vi "test TCX read (installed 71).vi"() -> ()   [LabVIEW 2011] (continued)
tensions></Trackpoint><Trackpoint><Time>2008-03-03T23:09:45Z</Time><Position><LatitudeDegrees>35.861013</LatitudeDegrees><LongitudeDegrees>-78.894979</LongitudeDegrees></Position><AltitudeMeters>65.026</AltitudeMeters><DistanceMeters>13506.518</DistanceMeters><Cadence>82</Cadence><Extensions><TPX xmlns=\"http://www.garmin.com/xmlschemas/ActivityExtension/v2\"><Watts>176</Watts></TPX></Extensions></Trackpoint><Trackpoint><Time>2008-03-03T23:09:46Z</Time><Position><LatitudeDegrees>35.861010</LatitudeDegrees><LongitudeDegrees>-78.895077</LongitudeDegrees></Position><AltitudeMeters>65.988</AltitudeMeters><DistanceMeters>13515.292</DistanceMeters><Cadence>82</Cadence><Extensions><TPX xmlns=\"http://www.garmin.com/xmlschemas/ActivityExtension/v2\"><Watts>178</Watts></TPX></Extensions></Trackpoint><Trackpoint><Time>2008-03-03T23:09:47Z</Time><Position><LatitudeDegrees>35.861009</LatitudeDegrees><LongitudeDegrees>-78.895172</LongitudeDegrees></Position><AltitudeMeters>65.988</AltitudeMeters><DistanceMeters>13523.903</DistanceMeters><Cadence>79</Cadence><Extensions><TPX xmlns=\"http://www.garmin.com/xmlschemas/ActivityExtension/v2\"><Watts>351</Watts></TPX></Extensions></Trackpoint><Trackpoint><Time>2008-03-03T23:09:48Z</Time><Position><LatitudeDegrees>35.861007</LatitudeDegrees><LongitudeDegrees>-78.895264</LongitudeDegrees></Position><AltitudeMeters>66.468</AltitudeMeters><DistanceMeters>13532.188</DistanceMeters><Cadence>78</Cadence><Extensions><TPX xmlns=\"http://www.garmin.com/xmlschemas/ActivityExtension/v2\"><Watts>435</Watts></TPX></Extensions></Trackpoint><Trackpoint><Time>2008-03-03T23:09:49Z</Time><Position><LatitudeDegrees>35.861004</LatitudeDegrees><LongitudeDegrees>-78.895353</LongitudeDegrees></Position><AltitudeMeters>66.468</AltitudeMeters><DistanceMeters>13540.193</DistanceMeters><Cadence>74</Cadence><Extensions><TPX xmlns=\"http://www.garmin.com/xmlschemas/ActivityExtension/v2\"><Watts>444</Watts></TPX></Extensions></Trackpoint><Trackpoint><Time>2008-03-03T23:09:50Z</Time><Position><LatitudeDegrees>35.861000</LatitudeDegrees><LongitudeDegrees>-78.895439</LongitudeDegrees></Position><AltitudeMeters>67.430</AltitudeMeters><DistanceMeters>13547.961</DistanceMeters><Cadence>73</Cadence><Extensions><TPX xmlns=\"http://www.garmin.com/xmlschemas/ActivityExtension/v2\"><Watts>439</Watts></TPX></Extensions></Trackpoint><Trackpoint><Time>2008-03-03T23:09:51Z</Time><Position><LatitudeDegrees>35.860996</LatitudeDegrees><LongitudeDegrees>-78.895523</LongitudeDegrees></Position><AltitudeMeters>67.910</AltitudeMeters><DistanceMeters>13555.550</DistanceMeters><Cadence>71</Cadence><Extensions><TPX xmlns=\"http://www.garmin.com/xmlschemas/ActivityExtension/v2\"><Watts>436</Watts></TPX></Extensions></Trackpoint><Trackpoint><Time>2008-03-03T23:09:52Z</Time><Position><LatitudeDegrees>35.860994</LatitudeDegrees><LongitudeDegrees>-78.895604</LongitudeDegrees></Position><AltitudeMeters>68.391</AltitudeMeters><DistanceMeters>13562.899</DistanceMeters><Cadence>69</Cadence><Extensions><TPX xmlns=\"http://www.garmin.com/xmlschemas/ActivityExtension/v2\"><Watts>446</Watts></TPX></Extensions></Trackpoint><Trackpoint><Time>2008-03-03T23:09:53Z</Time><Position><LatitudeDegrees>35.860992</LatitudeDegrees><LongitudeDegrees>-78.895685</LongitudeDegrees></Position><AltitudeMeters>68.872</AltitudeMeters><DistanceMeters>13570.170</DistanceMeters><Cadence>69</Cadence><Extensions><TPX xmlns=\"http://www.garmin.com/xmlschemas/ActivityExtension/v2\"><Watts>446</Watts></TPX></Extensions></Trackpoint><Trackpoint><Time>2008-03-03T23:09:54Z</Time><Position><LatitudeDegrees>35.860991</LatitudeDegrees><LongitudeDegrees>-78.895764</LongitudeDegrees></Position><AltitudeMeters>68.872</AltitudeMeters><DistanceMeters>13577.373</DistanceMeters><Cadence>66</Cadence><Extensions><TPX xmlns=\"http://www.garmin.com/xmlschemas/ActivityExtension/v2\"><Watts>426</Watts></TPX></Extensions></Trackpoint><Trackpoint><Time>2008-03-03T23:09:55Z</Time><Position><LatitudeDegrees>35.860992</LatitudeDegrees><LongitudeDegrees>-78.895843</LongitudeDegrees></Position><AltitudeMeters>69.352</AltitudeMeters><DistanceMeters>13584.441</DistanceMeters><Cadence>66</Cadence><Extensions><TPX xmlns=\"http://www.garmin.com/xmlschemas/ActivityExtension/v2\"><Watts>423</Watts></TPX></Extensions></Trackpoint><Trackpoint><Time>2008-03-03T23:09:56Z</Time><Position><LatitudeDegrees>35.860994</LatitudeDegrees><LongitudeDegrees>-78.895919</LongitudeDegrees></Position><AltitudeMeters>69.352</AltitudeMeters><DistanceMeters>13591.366</DistanceMeters><Cadence>64</Cadence><Extensions><TPX xmlns=\"http://www.garmin.com/xmlschemas/ActivityExtension/v2\"><Watts>377</Watts></TPX></Extensions></Trackpoint><Trackpoint><Time>2008-03-03T23:09:57Z</Time><Position><LatitudeDegrees>35.860996</LatitudeDegrees><LongitudeDegrees>-78.895995</LongitudeDegrees></Position><AltitudeMeters>69.833</AltitudeMeters><DistanceMeters>13598.160</DistanceMeters><Cadence>63</Cadence><Extensions><TPX xmlns=\"http://www.garmin.com/xmlschemas/ActivityExtension/v2\"><Watts>379</Watts></TPX></Extensions></Trackpoint><Trackpoint><Time>2008-03-03T23:09:58Z</Time><Position><LatitudeDegrees>35.861001</LatitudeDegrees><LongitudeDegrees>-78.896070</LongitudeDegrees></Position><AltitudeMeters>70.794</AltitudeMeters><DistanceMeters>13604.948</DistanceMeters><Cadence>63</Cadence><Extensions><TPX xmlns=\"http://www.garmin.com/xmlschemas/ActivityExtension/v2\"><Watts>379</Watts></TPX></Extensions></Trackpoint><Trackpoint><Time>2008-03-03T23:09:59Z</Time><Position><LatitudeDegrees>35.861008</LatitudeDegrees><LongitudeDegrees>-78.896144</LongitudeDegrees></Position><AltitudeMeters>70.794</AltitudeMeters><DistanceMeters>13611.671</DistanceMeters><Cadence>62</Cadence><Extensions><TPX xmlns=\"http://www.garmin.com/xmlschemas/ActivityExtension/v2\"><Watts>421</Watts></TPX></Extensions></Trackpoint><Trackpoint><Time>2008-03-03T23:10:00Z</Time><Position><LatitudeDegrees>35.861015</LatitudeDegrees><LongitudeDegrees>-78.896216</LongitudeDegrees></Position><AltitudeMeters>71.275</AltitudeMeters><DistanceMeters>13618.257</DistanceMeters><Cadence>62</Cadence><Extensions><TPX xmlns=\"http://www.garmin.com/xmlschemas/ActivityExtension/v2\"><Watts>418</Watts></TPX></Extensions></Trackpoint><Trackpoint><Time>2008-03-03T23:10:01Z</Time><Position><LatitudeDegrees>35.861021</LatitudeDegrees><LongitudeDegrees>-78.896289</LongitudeDegrees></Position><AltitudeMeters>71.755</AltitudeMeters><DistanceMeters>13624.921</DistanceMeters><Cadence>62</Cadence><Extensions><TPX xmlns=\"http://www.garmin.com/xmlschemas/ActivityExtension/v2\"><Watts>394</Watts></TPX></Extensions></Trackpoint><Trackpoint><Time>2008-03-03T23:10:02Z</Time><Position><LatitudeDegrees>35.861026</LatitudeDegrees><LongitudeDegrees>-78.896364</LongitudeDegrees></Position><AltitudeMeters>72.236</AltitudeMeters><DistanceMeters>13631.681</DistanceMeters><Cadence>63</Cadence><Extensions><TPX xmlns=\"http://www.garmin.com/xmlschemas/ActivityExtension/v2\"><Watts>395</Watts></TPX></Extensions></Trackpoint><Trackpoint><Time>2008-03-03T23:10:03Z</Time><Position><LatitudeDegrees>35.861030</LatitudeDegrees><LongitudeDegrees>-78.896439</LongitudeDegrees></Position><AltitudeMeters>72.236</AltitudeMeters><DistanceMeters>13638.502</DistanceMeters><Cadence>64</Cadence><Extensions><TPX xmlns=\"http://www.garmin.com/xmlschemas/ActivityExtension/v2\"><Watts>400</Watts></TPX></Extensions></Trackpoint><Trackpoint><Time>2008-03-03T23:10:04Z</Time><Position><LatitudeDegrees>35.861034</LatitudeDegrees><LongitudeDegrees>-78.896516</LongitudeDegrees></Position><AltitudeMeters>72.717</AltitudeMeters><DistanceMeters>13645.401</DistanceMeters><Cadence>64</Cadence><Extensions><TPX xmlns=\"http://www.garmin.com/xmlschemas/ActivityExtension/v2\"><Watts>409</Watts></TPX></Extensions></Trackpoint><Trackpoint><Time>2008-03-03T23:10:05Z</Time><Position><LatitudeDegrees>35.861039</LatitudeDegrees><LongitudeDegrees>-78.896593</LongitudeDegrees></Position><AltitudeMeters>72.717</AltitudeMeters><DistanceMeters>13652.380</DistanceMeters><Cadence>64</Cadence><Extensions><TPX xmlns=\"http://www.garmin.com/xmlschemas/ActivityExtension/v2\"><Watts>411</Watts></TPX></Extensions></Trackpoint><Trackpoint><Time>2008-03-03T23:10:06Z</Time><Position><LatitudeDegrees>35.861044</LatitudeDegrees><LongitudeDegrees>-78.896670</LongitudeDegrees></Position><AltitudeMeters>72.717</AltitudeMeters><DistanceMeters>13659.413</DistanceMeters><Cadence>67</Cadence><Extensions><TPX xmlns=\"http://www.garmin.com/xmlschemas/ActivityExtension/v2\"><Watts>418</Watts></TPX></Extensions></Trackpoint><Trackpoint><Time>2008-03-03T23:10:07Z</Time><Position><LatitudeDegrees>35.861050</LatitudeDegrees><LongitudeDegrees>-78.896750</LongitudeDegrees></Position><AltitudeMeters>73.198</AltitudeMeters><DistanceMeters>13666.635</DistanceMeters><Cadence>67</Cadence><Extensions><TPX xmlns=\"http://www.garmin.com/xmlschemas/ActivityExtension/v2\"><Watts>404</Watts></TPX></Extensions></Trackpoint><Trackpoint><Time>2008-03-03T23:10:08Z</Time><Position><LatitudeDegrees>35.861056</LatitudeDegrees><LongitudeDegrees>-78.896830</LongitudeDegrees></Position><AltitudeMeters>73.678</AltitudeMeters><DistanceMeters>13673.963</DistanceMeters><Cadence>69</Cadence><Extensions><TPX xmlns=\"http://www.garmin.com/xmlschemas/ActivityExtension/v2\"><Watts>388</Watts></TPX></Extensions></Trackpoint><Trackpoint><Time>2008-03-03T23:10:09Z</Time><Position><LatitudeDegrees>35.861062</LatitudeDegrees><LongitudeDegrees>-78.896912</LongitudeDegrees></Position><AltitudeMeters>74.159</AltitudeMeters><DistanceMeters>13681.418</DistanceMeters><Cadence>70</Cadence><Extensions><TPX xmlns=\"http://www.garmin.com/xmlschemas/ActivityExtension/v2\"><Watts>386</Watts></TPX></Extensions></Trackpoint><Trackpoint><Time>2008-03-03T23:10:10Z</Time><Position><LatitudeDegrees>35.861070</LatitudeDegrees><LongitudeDegrees>-78.896996</LongitudeDegrees></Position><AltitudeMeters>74.640</AltitudeMeters><DistanceMeters>13689.080</DistanceMeters><Cadence>70</Cadence><Extensions><TPX xmlns=\"http://www.garmin.com/xmlschemas/ActivityExtension/v2\"><Watts>384</Watts></TPX></Extensions></Trackpoint><Trackpoint><Time>2008-03-03T23:10:11Z</Time><Position><LatitudeDegrees>35.861077</LatitudeDegrees><LongitudeDegrees>-78.897082</LongitudeDegrees></Position><AltitudeMeters>74.640</AltitudeMeters><DistanceMeters>13696.857</DistanceMeters><Cadence>72</Cadence><Extensions><TPX xmlns=\"http://www.garmin.com/xmlschemas/ActivityExtension/v2\"><Watts>388</Watts></TPX></Extensions></Trackpoint><Trackpoint><Time>2008-03-03T23:10:12Z</Time><Position><LatitudeDegrees>35.861085</LatitudeDegrees><LongitudeDegrees>-78.897170</LongitudeDegrees></Position><AltitudeMeters>75.120</AltitudeMeters><DistanceMeters>13704.818</DistanceMeters><Cadence>74</Cadence><Extensions><TPX xmlns=\"http://www.garmin.com/xmlschemas/ActivityExtension/v2\"><Watts>392</Watts></TPX></Extensions></Trackpoint><Trackpoint><Time>2008-03-03T23:10:13Z</Time><Position><LatitudeDegrees>35.861095</LatitudeDegrees><LongitudeDegrees>-78.897259</LongitudeDegrees></Position><AltitudeMeters>75.601</AltitudeMeters><DistanceMeters>13712.946</DistanceMeters><Cadence>76</Cadence><Extensions><TPX xmlns=\"http://www.garmin.com/xmlschemas/ActivityExtension/v2\"><Watts>393</Watts></TPX></Extensions></Trackpoint><Trackpoint><Time>2008-03-03T23:10:14Z</Time><Position><LatitudeDegrees>35.861106</LatitudeDegrees><LongitudeDegrees>-78.897348</LongitudeDegrees></Position><AltitudeMeters>75.120</AltitudeMeters><DistanceMeters>13721.106</DistanceMeters><Cadence>75</Cadence><Extensions><TPX xmlns=\"http://www.garmin.com/xmlschemas/ActivityExtension/v2\"><Watts>364</Watts></TPX></Extensions></Trackpoint><Trackpoint><Time>2008-03-03T23:10:15Z</Time><Position><LatitudeDegrees>35.861116</LatitudeDegrees><LongitudeDegrees>-78.897436</LongitudeDegrees></Position><AltitudeMeters>75.601</AltitudeMeters><DistanceMeters>13729.120</DistanceMeters><Cadence>74</Cadence><Extensions><TPX xmlns=\"http://www.garmin.com/xmlschemas/ActivityExtension/v2\"><Watts>233</Watts></TPX></Extensions></Trackpoint><Trackpoint><Time>2008-03-03T23:10:16Z</Time><Position><LatitudeDegrees>35.861124</LatitudeDegrees><LongitudeDegrees>-78.897522</LongitudeDegrees></Position><AltitudeMeters>75.601</AltitudeMeters><DistanceMeters>13736.914</DistanceMeters><Cadence>72</Cadence><Extensions><TPX xmlns=\"http://www.garmin.com/xmlschemas/ActivityExtension/v2\"><Watts>107</Watts></TPX></Extensions></Trackpoint><Trackpoint><Time>2008-03-03T23:10:17Z</Time><Position><LatitudeDegrees>35.861136</LatitudeDegrees><LongitudeDegrees>-78.897604</LongitudeDegrees></Position><AltitudeMeters>75.601</AltitudeMeters><DistanceMeters>13744.367</DistanceMeters><Cadence>69</Cadence><Extensions><TPX xmlns=\"http://www.garmin.com/xmlschemas/ActivityExtension/v2\"><Watts>52</Watts></TPX></Extensions></Trackpoint><Trackpoint><Time>2008-03-03T23:10:18Z</Time><Position><LatitudeDegrees>35.861166</LatitudeDegrees><LongitudeDegrees>-78.897671</LongitudeDegrees></Position><AltitudeMeters>76.081</AltitudeMeters><DistanceMeters>13751.099</DistanceMeters><Cadence>68</Cadence><Extensions><TPX xmlns=\"http://www.garmin.com/xmlschemas/ActivityExtension/v2\"><Watts>52</Watts></TPX></Extensions></Trackpoint><Trackpoint><Time>2008-03-03T23:10:19Z</Time><Position><LatitudeDegrees>35.861226</LatitudeDegrees><LongitudeDegrees>-78.897707</LongitudeDegrees></Position><AltitudeMeters>76.562</AltitudeMeters><DistanceMeters>13758.359</DistanceMeters><Cadence>63</Cadence><Extensions><TPX xmlns=\"http://www.garmin.com/xmlschemas/ActivityExtension/v2\"><Watts>60</Watts></TPX></Extensions></Trackpoint><Trackpoint><Time>2008-03-03T23:10:20Z</Time><Position><LatitudeDegrees>35.861288</LatitudeDegrees><LongitudeDegrees>-78.897691</LongitudeDegrees></Position><AltitudeMeters>77.043</AltitudeMeters><DistanceMeters>13765.466</DistanceMeters><Cadence>63</Cadence><Extensions><TPX xmlns=\"http://www.garmin.com/xmlschemas/ActivityExtension/v2\"><Watts>59</Watts></TPX></Extensions></Trackpoint><Trackpoint><Time>2008-03-03T23:10:21Z</Time><Position><LatitudeDegrees>35.861350</LatitudeDegrees><LongitudeDegrees>-78.897655</LongitudeDegrees></Position><AltitudeMeters>77.043</AltitudeMeters><DistanceMeters>13773.082</DistanceMeters><Cadence>65</Cadence><Extensions><TPX xmlns=\"http://www.garmin.com/xmlschemas/ActivityExtension/v2\"><Watts>377</Watts></TPX></Extensions></Trackpoint><Trackpoint><Time>2008-03-03T23:10:22Z</Time><Position><LatitudeDegrees>35.861415</LatitudeDegrees><LongitudeDegrees>-78.897617</LongitudeDegrees></Position><AltitudeMeters>77.523</AltitudeMeters><DistanceMeters>13781.167</DistanceMeters><Cadence>68</Cadence><Extensions><TPX xmlns=\"http://www.garmin.com/xmlschemas/ActivityExtension/v2\"><Watts>429</Watts></TPX></Extensions></Trackpoint><Trackpoint><Time>2008-03-03T23:10:23Z</Time><Position><LatitudeDegrees>35.861477</LatitudeDegrees><LongitudeDegrees>-78.897576</LongitudeDegrees></Position><AltitudeMeters>77.523</AltitudeMeters><DistanceMeters>13788.905</DistanceMeters><Cadence>70</Cadence><Extensions><TPX xmlns=\"http://www.garmin.com/xmlschemas/ActivityExtension/v2\"><Watts>456</Watts></TPX></Extensions></Trackpoint><Trackpoint><Time>2008-03-03T23:10:24Z</Time><Position><LatitudeDegrees>35.861541</LatitudeDegrees><LongitudeDegrees>-78.897533</LongitudeDegrees></Position><AltitudeMeters>78.004</AltitudeMeters><DistanceMeters>13797.001</DistanceMeters><Cadence>71</Cadence><Extensions><TPX xmlns=\"http://www.garmin.com/xmlschemas/ActivityExtension/v2\"><Watts>430</Watts></TPX></Extensions></Trackpoint><Trackpoint><Time>2008-03-03T23:10:25Z</Time><Position><LatitudeDegrees>35.861605</LatitudeDegrees><LongitudeDegrees>-78.897493</LongitudeDegrees></Position><AltitudeMeters>78.004</AltitudeMeters><DistanceMeters>13804.948</DistanceMeters><Cadence>73</Cadence><Extensions><TPX xmlns=\"http://www.garmin.com/xmlschemas/ActivityExtension/v2\"><Watts>403</Watts></TPX></Extensions></Trackpoint><Trackpoint><Time>2008-03-03T23:10:26Z</Time><Position><LatitudeDegrees>35.861668</LatitudeDegrees><LongitudeDegrees>-78.897454</LongitudeDegrees></Position><AltitudeMeters>78.485</AltitudeMeters><DistanceMeters>13812.879</DistanceMeters><Cadence>73</Cadence><Extensions><TPX xmlns=\"http://www.garmin.com/xmlschemas/ActivityExtension/v2\"><Watts>345</Watts></TPX></Extensions></Trackpoint><Trackpoint><Time>2008-03-03T23:10:27Z</Time><Position><LatitudeDegrees>35.861733</LatitudeDegrees><LongitudeDegrees>-78.897415</LongitudeDegrees></Position><AltitudeMeters>78.004</AltitudeMeters><DistanceMeters>13820.811</DistanceMeters><Cadence>72</Cadence><Extensions><TPX xmlns=\"http://www.garmin.com/xmlschemas/ActivityExtension/v2\"><Watts>316</Watts></TPX></Extensions></Trackpoint><Trackpoint><Time>2008-03-03T23:10:28Z</Time><Position><LatitudeDegrees>35.861798</LatitudeDegrees><LongitudeDegrees>-78.897377</LongitudeDegrees></Position><AltitudeMeters>78.485</AltitudeMeters><DistanceMeters>13828.832</DistanceMeters><Cadence>72</Cadence><Extensions><TPX xmlns=\"http://www.garmin.com/xmlschemas/ActivityExtension/v2\"><Watts>292</Watts></TPX></Extensions></Trackpoint><Trackpoint><Time>2008-03-03T23:10:29Z</Time><Position><LatitudeDegrees>35.861861</LatitudeDegrees><LongitudeDegrees>-78.897341</LongitudeDegrees></Position><AltitudeMeters>78.965</AltitudeMeters><DistanceMeters>13836.527</DistanceMeters><Cadence>72</Cadence><Extensions><TPX xmlns=\"http://www.garmin.com/xmlschemas/ActivityExtension/v2\"><Watts>274</Watts></TPX></Extensions></Trackpoint><Trackpoint><Time>2008-03-03T23:10:30Z</Time><Position><LatitudeDegrees>35.861924</LatitudeDegrees><LongitudeDegrees>-78.897309</LongitudeDegrees></Position><AltitudeMeters>79.446</AltitudeMeters><DistanceMeters>13844.088</DistanceMeters><Cadence>72</Cadence><Extensions><TPX xmlns=\"http://www.garmin.com/xmlschemas/ActivityExtension/v2\"><Watts>276</Watts></TPX></Extensions></Trackpoint><Trackpoint><Time>2008-03-03T23:10:31Z</Time><Position><LatitudeDegrees>35.861985</LatitudeDegrees><LongitudeDegrees>-78.897277</LongitudeDegrees></Position><AltitudeMeters>79.446</AltitudeMeters><DistanceMeters>13851.475</DistanceMeters><Cadence>70</Cadence><Extensions><TPX xmlns=\"http://www.garmin.com/xmlschemas/ActivityExtension/v2\"><Watts>273</Watts></TPX></Extensions></Trackpoint><Trackpoint><Time>2008-03-03T23:10:32Z</Time><Position><LatitudeDegrees>35.862050</LatitudeDegrees><LongitudeDegrees>-78.897251</LongitudeDegrees></Position><AltitudeMeters>79.446</AltitudeMeters><DistanceMeters>13859.048</DistanceMeters><Cadence>70</Cadence><Extensions><TPX xmlns=\"http://www.garmin.com/xmlschemas/ActivityExtension/v2\"><Watts>271</Watts></TPX></Extensions></Trackpoint><Trackpoint><Time>2008-03-03T23:10:33Z</Time><Position><LatitudeDegrees>35.862113</LatitudeDegrees><LongitudeDegrees>-78.897226</LongitudeDegrees></Position><AltitudeMeters>79.446</AltitudeMeters><DistanceMeters>13866.438</DistanceMeters><Cadence>69</Cadence><Extensions><TPX xmlns=\"http://www.garmin.com/xmlschemas/ActivityExtension/v2\"><Watts>260</Watts></TPX></Extensions></Trackpoint><Trackpoint><Time>2008-03-03T23:10:34Z</Time><Position><LatitudeDegrees>35.862177</LatitudeDegrees><LongitudeDegrees>-78.897201</LongitudeDegrees></Position><AltitudeMeters>79.927</AltitudeMeters><DistanceMeters>13873.806</DistanceMeters><Cadence>68</Cadence><Extensions><TPX xmlns=\"http://www.garmin.com/xmlschemas/ActivityExtension/v2\"><Watts>233</Watts></TPX></Extensions></Trackpoint><Trackpoint><Time>2008-03-03T23:10:35Z</Time><Position><LatitudeDegrees>35.862241</LatitudeDegrees><LongitudeDegrees>-78.897177</LongitudeDegrees></Position><AltitudeMeters>79.927</AltitudeMeters><DistanceMeters>13881.198</DistanceMeters><Cadence>68</Cadence><Extensions><TPX xmlns=\"http://www.garmin.com/xmlschemas/ActivityExtension/v2\"><Watts>232</Watts></TPX></Extensions></Trackpoint><Trackpoint><Time>2008-03-03T23:10:36Z</Time><Position><LatitudeDegrees>35.862304</LatitudeDegrees><LongitudeDegrees>-78.897157</LongitudeDegrees></Position><AltitudeMeters>79.927</AltitudeMeters><DistanceMeters>13888.406</DistanceMeters><Cadence>67</Cadence><Extensions><TPX xmlns=\"http://www.garmin.com/xmlschemas/ActivityExtension/v2\"><Watts>164</Watts></TPX></Extensions></Trackpoint><Trackpoint><Time>2008-03-03T23:10:37Z</Time><Position><LatitudeDegrees>35.862367</LatitudeDegrees><LongitudeDegrees>-78.897137</LongitudeDegrees></Position><AltitudeMeters>80.407</AltitudeMeters><DistanceMeters>13895.671</DistanceMeters><Cadence>66</Cadence><Extensions><TPX xmlns=\"http://www.garmin.com/xmlschemas/ActivityExtension/v2\"><Watts>164</Watts></TPX></Extensions></Trackpoint><Trackpoint><Time>2008-03-03T23:10:38Z</Time><Position><LatitudeDegrees>35.862429</LatitudeDegrees><LongitudeDegrees>-78.897119</LongitudeDegrees></Position><AltitudeMeters>80.407</AltitudeMeters><DistanceMeters>13902.797</DistanceMeters><Cadence>66</Cadence><Extensions><TPX xmlns=\"http://www.garmin.com/xmlschemas/ActivityExtension/v2\"><Watts>171</Watts></TPX></Extensions></Trackpoint><Trackpoint><Time>2008-03-03T23:10:39Z</Time><Position><LatitudeDegrees>35.862493</LatitudeDegrees><LongitudeDegrees>-78.897101</LongitudeDegrees></Position><AltitudeMeters>80.407</AltitudeMeters><DistanceMeters>13910.059</DistanceMeters><Cadence>66</Cadence><Extensions><TPX xmlns=\"http://www.garmin.com/xmlschemas/ActivityExtension/v2\"><Watts>173</Watts></TPX></Extensions></Trackpoint><Trackpoint><Time>2008-03-03T23:10:40Z</Time><Position><LatitudeDegrees>35.862555</LatitudeDegrees><LongitudeDegrees>-78.897088</LongitudeDegrees></Position><AltitudeMeters>80.407</AltitudeMeters><DistanceMeters>13917.023</DistanceMeters><Cadence>66</Cadence><Extensions><TPX xmlns=\"http://www.garmin.com/xmlschemas/ActivityExtension/v2\"><Watts>170</Watts></TPX></Extensions></Trackpoint><Trackpoint><Time>2008-03-03T23:10:41Z</Time><Position><LatitudeDegrees>35.862619</LatitudeDegrees><LongitudeDegrees>-78.897075</LongitudeDegrees></Position><AltitudeMeters>80.407</AltitudeMeters><DistanceMeters>13924.162</DistanceMeters><Cadence>66</Cadence><Extensions><TPX xmlns=\"http://www.garmin.com/xmlschemas/ActivityExtension/v2\"><Watts>163</Watts></TPX></Extensions></Trackpoint><Trackpoint><Time>2008-03-03T23:10:42Z</Time><Position><LatitudeDegrees>35.862684</LatitudeDegrees><LongitudeDegrees>-78.897063</LongitudeDegrees></Position><AltitudeMeters>80.888</AltitudeMeters><DistanceMeters>13931.451</DistanceMeters><Cadence>66</Cadence><Extensions><TPX xmlns=\"http://www.garmin.com/xmlschemas/ActivityExtension/v2\"><Watts>165</Watts></TPX></Extensions></Trackpoint><Trackpoint><Time>2008-03-03T23:10:43Z</Time><Position><LatitudeDegrees>35.862747</LatitudeDegrees><LongitudeDegrees>-78.897053</LongitudeDegrees></Position><AltitudeMeters>80.888</AltitudeMeters><DistanceMeters>13938.466</DistanceMeters><Cadence>65</Cadence><Extensions><TPX xmlns=\"http://www.garmin.com/xmlschemas/ActivityExtension/v2\"><Watts>145</Watts></TPX></Extensions></Trackpoint><Trackpoint><Time>2008-03-03T23:10:44Z</Time><Position><LatitudeDegrees>35.862810</LatitudeDegrees><LongitudeDegrees>-78.897044</LongitudeDegrees></Position><AltitudeMeters>80.888</AltitudeMeters><DistanceMeters>13945.525</DistanceMeters><Cadence>65</Cadence><Extensions><TPX xmlns=\"http://www.garmin.com/xmlschemas/ActivityExtension/v2\"><Watts>149</Watts></TPX></Extensions></Trackpoint><Trackpoint><Time>2008-03-03T23:10:45Z</Time><Position><LatitudeDegrees>35.862874</LatitudeDegrees><LongitudeDegrees>-78.897035</LongitudeDegrees></Position><AltitudeMeters>81.369</AltitudeMeters><DistanceMeters>13952.661</DistanceMeters><Cadence>65</Cadence><Extensions><TPX xmlns=\"http://www.garmin.com/xmlschemas/ActivityExtension/v2\"><Watts>137</Watts></TPX></Extensions></Trackpoint><Trackpoint><Time>2008-03-03T23:10:46Z</Time><Position><LatitudeDegrees>35.862936</LatitudeDegrees><LongitudeDegrees>-78.897027</LongitudeDegrees></Position><AltitudeMeters>81.369</AltitudeMeters><DistanceMeters>13959.629</DistanceMeters><Cadence>64</Cadence><Extensions><TPX xmlns=\"http://www.garmin.com/xmlschemas/ActivityExtension/v2\"><Watts>136</Watts></TPX></Extensions></Trackpoint><Trackpoint><Time>2008-03-03T23:10:47Z</Time><Position><LatitudeDegrees>35.862997</LatitudeDegrees><LongitudeDegrees>-78.897017</LongitudeDegrees></Position><AltitudeMeters>81.369</AltitudeMeters><DistanceMeters>13966.494</DistanceMeters><Cadence>65</Cadence><Extensions><TPX xmlns=\"http://www.garmin.com/xmlschemas/ActivityExtension/v2\"><Watts>138</Watts></TPX></Extensions></Trackpoint><Trackpoint><Time>2008-03-03T23:10:48Z</Time><Position><LatitudeDegrees>35.863060</LatitudeDegrees><LongitudeDegrees>-78.897006</LongitudeDegrees></Position><AltitudeMeters>81.369</AltitudeMeters><DistanceMeters>13973.530</DistanceMeters><Cadence>65</Cadence><Extensions><TPX xmlns=\"http://www.garmin.com/xmlschemas/ActivityExtension/v2\"><Watts>130</Watts></TPX></Extensions></Trackpoint><Trackpoint><Time>2008-03-03T23:10:49Z</Time><Position><LatitudeDegrees>35.863124</LatitudeDegrees><LongitudeDegrees>-78.896995</LongitudeDegrees></Position><AltitudeMeters>81.369</AltitudeMeters><DistanceMeters>13980.699</DistanceMeters><Cadence>65</Cadence><Extensions><TPX xmlns=\"http://www.garmin.com/xmlschemas/ActivityExtension/v2\"><Watts>126</Watts></TPX></Extensions></Trackpoint><Trackpoint><Time>2008-03-03T23:10:50Z</Time><Position><LatitudeDegrees>35.863189</LatitudeDegrees><LongitudeDegrees>-78.896986</LongitudeDegrees></Position><AltitudeMeters>81.849</AltitudeMeters><DistanceMeters>13987.968</DistanceMeters><Cadence>65</Cadence><Extensions><TPX xmlns=\"http://www.garmin.com/xmlschemas/ActivityExtension/v2\"><Watts>125</Watts></TPX></Extensions></Trackpoint><Trackpoint><Time>2008-03-03T23:10:51Z</Time><Position><LatitudeDegrees>35.863253</LatitudeDegrees><LongitudeDegrees>-78.896977</LongitudeDegrees></Position><AltitudeMeters>81.849</AltitudeMeters><DistanceMeters>13995.102</DistanceMeters><Cadence>65</Cadence><Extensions><TPX xmlns=\"http://www.garmin.com/xmlschemas/ActivityExtension/v2\"><Watts>105</Watts></TPX></Extensions></Trackpoint><Trackpoint><Time>2008-03-03T23:10:52Z</Time><Position><LatitudeDegrees>35.863315</LatitudeDegrees><LongitudeDegrees>-78.896968</LongitudeDegrees></Position><AltitudeMeters>81.849</AltitudeMeters><DistanceMeters>14001.995</DistanceMeters><Cadence>65</Cadence><Extensions><TPX xmlns=\"http://www.garmin.com/xmlschemas/ActivityExtension/v2\"><Watts>106</Watts></TPX></Extensions></Trackpoint><Trackpoint><Time>2008-03-03T23:10:53Z</Time><Position><LatitudeDegrees>35.863377</LatitudeDegrees><LongitudeDegrees>-78.896958</LongitudeDegrees></Position><AltitudeMeters>82.330</AltitudeMeters><DistanceMeters>14008.998</DistanceMeters><Cadence>65</Cadence><Extensions><TPX xmlns=\"http://www.garmin.com/xmlschemas/ActivityExtension/v2\"><Watts>99</Watts></TPX></Extensions></Trackpoint><Trackpoint><Time>2008-03-03T23:10:54Z</Time><Position><LatitudeDegrees>35.863440</LatitudeDegrees><LongitudeDegrees>-78.896948</LongitudeDegrees></Position><AltitudeMeters>82.330</AltitudeMeters><DistanceMeters>14015.998</DistanceMeters><Cadence>65</Cadence><Extensions><TPX xmlns=\"http://www.garmin.com/xmlschemas/ActivityExtension/v2\"><Watts>101</Watts></TPX></Extensions></Trackpoint><Trackpoint><Time>2008-03-03T23:10:55Z</Time><Position><LatitudeDegrees>35.863503</LatitudeDegrees><LongitudeDegrees>-78.896938</LongitudeDegrees></Position><AltitudeMeters>82.330</AltitudeMeters><DistanceMeters>14023.096</DistanceMeters><Cadence>65</Cadence><Extensions><TPX xmlns=\"http://www.garmin.com/xmlschemas/ActivityExtension/v2\"><Watts>100</Watts></TPX></Extensions></Trackpoint><Trackpoint><Time>2008-03-03T23:10:56Z</Time><Position><LatitudeDegrees>35.863566</LatitudeDegrees><LongitudeDegrees>-78.896934</LongitudeDegrees></Position><AltitudeMeters>82.330</AltitudeMeters><DistanceMeters>14030.051</DistanceMeters><Cadence>65</Cadence><Extensions><TPX xmlns=\"http://www.garmin.com/xmlschemas/ActivityExtension/v2\"><Watts>106</Watts></TPX></Extensions></Trackpoint><Trackpoint><Time>2008-03-03T23:10:57Z</Time><Position><LatitudeDegrees>35.863627</LatitudeDegrees><LongitudeDegrees>-78.896940</LongitudeDegrees></Position><AltitudeMeters>82.811</AltitudeMeters><DistanceMeters>14036.868</DistanceMeters><Cadence>64</Cadence><Extensions><TPX xmlns=\"http://www.garmin.com/xmlschemas/ActivityExtension/v2\"><Watts>106</Watts></TPX></Extensions></Trackpoint><Trackpoint><Time>2008-03-03T23:10:58Z</Time><Position><LatitudeDegrees>35.863685</LatitudeDegrees><LongitudeDegrees>-78.896964</LongitudeDegrees></Position><AltitudeMeters>83.291</AltitudeMeters><DistanceMeters>14043.521</DistanceMeters><Cadence>62</Cadence><Extensions><TPX xmlns=\"http://www.garmin.com/xmlschemas/ActivityExtension/v2\"><Watts>104</Watts></TPX></Extensions></Trackpoint><Trackpoint><Time>2008-03-03T23:10:59Z</Time><Position><LatitudeDegrees>35.863732</LatitudeDegrees><LongitudeDegrees>-78.897007</LongitudeDegrees></Position><AltitudeMeters>82.811</AltitudeMeters><DistanceMeters>14049.984</DistanceMeters><Cadence>62</Cadence><Extensions><TPX xmlns=\"http://www.garmin.com/xmlschemas/ActivityExtension/v2\"><Watts>102</Watts></TPX></Extensions></Trackpoint><Trackpoint><Time>2008-03-03T23:11:00Z</Time><Position><LatitudeDegrees>35.863767</LatitudeDegrees><LongitudeDegrees>-78.897066</LongitudeDegrees></Position><AltitudeMeters>83.291</AltitudeMeters><DistanceMeters>14056.616</DistanceMeters><Cadence>62</Cadence><Extensions><TPX xmlns=\"http://www.garmin.com/xmlschemas/ActivityExtension/v2\"><Watts>97</Watts></TPX></Extensions></Trackpoint><Trackpoint><Time>2008-03-03T23:11:01Z</Time><Position><LatitudeDegrees>35.863788</LatitudeDegrees><LongitudeDegrees>-78.897137</LongitudeDegrees></Position><AltitudeMeters>83.291</AltitudeMeters><DistanceMeters>14063.417</DistanceMeters><Cadence>64</Cadence><Extensions><TPX xmlns=\"http://www.garmin.com/xmlschemas/ActivityExtension/v2\"><Watts>92</Watts></TPX></Extensions></Trackpoint><Trackpoint><Time>2008-03-03T23:11:02Z</Time><Position><LatitudeDegrees>35.863794</LatitudeDegrees><LongitudeDegrees>-78.897215</LongitudeDegrees></Position><AltitudeMeters>82.811</AltitudeMeters><DistanceMeters>14070.526</DistanceMeters><Cadence>64</Cadence><Extensions><TPX xmlns=\"http://www.garmin.com/xmlschemas/ActivityExtension/v2\"><Watts>92</Watts></TPX></Extensions></Trackpoint><Trackpoint><Time>2008-03-03T23:11:03Z</Time><Position><LatitudeDegrees>35.863787</LatitudeDegrees><LongitudeDegrees>-78.897296</LongitudeDegrees></Position><AltitudeMeters>83.291</AltitudeMeters><DistanceMeters>14077.847</DistanceMeters><Cadence>66</Cadence><Extensions><TPX xmlns=\"http://www.garmin.com/xmlschemas/ActivityExtension/v2\"><Watts>87</Watts></TPX></Extensions></Trackpoint><Trackpoint><Time>2008-03-03T23:11:04Z</Time><Position><LatitudeDegrees>35.863773</LatitudeDegrees><LongitudeDegrees>-78.897378</LongitudeDegrees></Position><AltitudeMeters>82.811</AltitudeMeters><DistanceMeters>14085.448</DistanceMeters><Cadence>68</Cadence><Extensions><TPX xmlns=\"http://www.garmin.com/xmlschemas/ActivityExtension/v2\"><Watts>87</Watts></TPX></Extensions></Trackpoint><Trackpoint><Time>2008-03-03T23:11:05Z</Time><Position><LatitudeDegrees>35.863759</LatitudeDegrees><LongitudeDegrees>-78.897462</LongitudeDegrees></Position><AltitudeMeters>82.811</AltitudeMeters><DistanceMeters>14093.145</DistanceMeters><Cadence>70</Cadence><Extensions><TPX xmlns=\"http://www.garmin.com/xmlschemas/ActivityExtension/v2\"><Watts>86</Watts></TPX></Extensions></Trackpoint><Trackpoint><Time>2008-03-03T23:11:06Z</Time><Position><LatitudeDegrees>35.863746</LatitudeDegrees><LongitudeDegrees>-78.897548</LongitudeDegrees></Position><AltitudeMeters>82.811</AltitudeMeters><DistanceMeters>14101.066</DistanceMeters><Cadence>72</Cadence><Extensions><TPX xmlns=\"http://www.garmin.com/xmlschemas/ActivityExtension/v2\"><Watts>86</Watts></TPX></Extensions></Trackpoint><Trackpoint><Time>2008-03-03T23:11:07Z</Time><Position><LatitudeDegrees>35.863735</LatitudeDegrees><LongitudeDegrees>-78.897635</LongitudeDegrees></Position><AltitudeMeters>82.811</AltitudeMeters><DistanceMeters>14109.060</DistanceMeters><Cadence>72</Cadence><Extensions><TPX xmlns=\"http://www.garmin.com/xmlschemas/ActivityExtension/v2\"><Watts>86</Watts></TPX></Extensions></Trackpoint><Trackpoint><Time>2008-03-03T23:11:08Z</Time><Position><LatitudeDegrees>35.863720</LatitudeDegrees><LongitudeDegrees>-78.897725</LongitudeDegrees></Position><AltitudeMeters>82.811</AltitudeMeters><DistanceMeters>14117.366</DistanceMeters><Cadence>74</Cadence><Extensions><TPX xmlns=\"http://www.garmin.com/xmlschemas/ActivityExtension/v2\"><Watts>80</Watts></TPX></Extensions></Trackpoint><Trackpoint><Time>2008-03-03T23:11:09Z</Time><Position><LatitudeDegrees>35.863704</LatitudeDegrees><LongitudeDegrees>-78.897817</LongitudeDegrees></Position><AltitudeMeters>82.330</AltitudeMeters><DistanceMeters>14125.814</DistanceMeters><Cadence>76</Cadence><Extensions><TPX xmlns=\"http://www.garmin.com/xmlschemas/ActivityExtension/v2\"><Watts>82</Watts></TPX></Extensions></Trackpoint><Trackpoint><Time>2008-03-03T23:11:10Z</Time><Position><LatitudeDegrees>35.863692</LatitudeDegrees><LongitudeDegrees>-78.897911</LongitudeDegrees></Position><AltitudeMeters>82.330</AltitudeMeters><DistanceMeters>14134.484</DistanceMeters><Cadence>76</Cadence><Extensions><TPX xmlns=\"http://www.garmin.com/xmlschemas/ActivityExtension/v2\"><Watts>70</Watts></TPX></Extensions></Trackpoint><Trackpoint><Time>2008-03-03T23:11:11Z</Time><Position><LatitudeDegrees>35.863680</LatitudeDegrees><LongitudeDegrees>-78.898007</LongitudeDegrees></Position><AltitudeMeters>82.330</AltitudeMeters><DistanceMeters>14143.236</DistanceMeters><Cadence>70</Cadence><Extensions><TPX xmlns=\"http://www.garmin.com/xmlschemas/ActivityExtension/v2\"><Watts>75</Watts></TPX></Extensions></Trackpoint><Trackpoint><Time>2008-03-03T23:11:12Z</Time><Position><LatitudeDegrees>35.863664</LatitudeDegrees><LongitudeDegrees>-78.898104</LongitudeDegrees></Position><AltitudeMeters>81.849</AltitudeMeters><DistanceMeters>14152.142</DistanceMeters><Cadence>71</Cadence><Extensions><TPX xmlns=\"http://www.garmin.com/xmlschemas/ActivityExtension/v2\"><Watts>74</Watts></TPX></Extensions></Trackpoint><Trackpoint><Time>2008-03-03T23:11:13Z</Time><Position><LatitudeDegrees>35.863646</LatitudeDegrees><LongitudeDegrees>-78.898202</LongitudeDegrees></Position><AltitudeMeters>81.849</AltitudeMeters><DistanceMeters>14161.266</DistanceMeters><Cadence>71</Cadence><Extensions><TPX xmlns=\"http://www.garmin.com/xmlschemas/ActivityExtension/v2\"><Watts>77</Watts></TPX></Extensions></Trackpoint><Trackpoint><Time>2008-03-03T23:11:14Z</Time><Position><LatitudeDegrees>35.863626</LatitudeDegrees><LongitudeDegrees>-78.898301</LongitudeDegrees></Position><AltitudeMeters>81.849</AltitudeMeters><DistanceMeters>14170.506</DistanceMeters><Cadence>72</Cadence><Extensions><TPX xmlns=\"http://www.garmin.com/xmlschemas/ActivityExtension/v2\"><Watts>81</Watts></TPX></Extensions></Trackpoint><Trackpoint><Time>2008-03-03T23:11:15Z</Time><Position><LatitudeDegrees>35.863605</LatitudeDegrees><LongitudeDegrees>-78.898401</LongitudeDegrees></Position><AltitudeMeters>81.849</AltitudeMeters><DistanceMeters>14179.803</DistanceMeters><Cadence>73</Cadence><Extensions><TPX xmlns=\"http://www.garmin.com/xmlschemas/ActivityExtension/v2\"><Watts>84</Watts></TPX></Extensions></Trackpoint><Trackpoint><Time>2008-03-03T23:11:16Z</Time><Position><LatitudeDegrees>35.863579</LatitudeDegrees><LongitudeDegrees>-78.898503</LongitudeDegrees></Position><AltitudeMeters>81.369</AltitudeMeters><DistanceMeters>14189.492</DistanceMeters><Cadence>74</Cadence><Extensions><TPX xmlns=\"http://www.garmin.com/xmlschemas/ActivityExtension/v2\"><Watts>79</Watts></TPX></Extensions></Trackpoint><Trackpoint><Time>2008-03-03T23:11:17Z</Time><Position><LatitudeDegrees>35.863559</LatitudeDegrees><LongitudeDegrees>-78.898605</LongitudeDegrees></Position><AltitudeMeters>80.888</AltitudeMeters><DistanceMeters>14198.928</DistanceMeters><Cadence>75</Cadence><Extensions><TPX xmlns=\"http://www.garmin.com/xmlschemas/ActivityExtension/v2\"><Watts>87</Watts></TPX></Extensions></Trackpoint><Trackpoint><Time>2008-03-03T23:11:18Z</Time><Position><LatitudeDegrees>35.863544</LatitudeDegrees><LongitudeDegrees>-78.898709</LongitudeDegrees></Position><AltitudeMeters>80.407</AltitudeMeters><DistanceMeters>14208.516</DistanceMeters><Cadence>75</Cadence><Extensions><TPX xmlns=\"http://www.garmin.com/xmlschemas/ActivityExtension/v2\"><Watts>67</Watts></TPX></Extensions></Trackpoint><Trackpoint><Time>2008-03-03T23:11:19Z</Time><Position><LatitudeDegrees>35.863529</LatitudeDegrees><LongitudeDegrees>-78.898816</LongitudeDegrees></Position><AltitudeMeters>79.927</AltitudeMeters><DistanceMeters>14218.289</DistanceMeters><Cadence>75</Cadence><Extensions><TPX xmlns=\"http://www.garmin.com/xmlschemas/ActivityExtension/v2\"><Watts>66</Watts></TPX></Extensions></Trackpoint><Trackpoint><Time>2008-03-03T23:11:20Z</Time><Position><LatitudeDegrees>35.863513</LatitudeDegrees><LongitudeDegrees>-78.898923</LongitudeDegrees></Position><AltitudeMeters>79.927</AltitudeMeters><DistanceMeters>14228.184</DistanceMeters><Cadence>75</Cadence><Extensions><TPX xmlns=\"http://www.garmin.com/xmlschemas/ActivityExtension/v2\"><Watts>61</Watts></TPX></Extensions></Trackpoint><Trackpoint><Time>2008-03-03T23:11:21Z</Time><Position><LatitudeDegrees>35.863494</LatitudeDegrees><LongitudeDegrees>-78.899034</LongitudeDegrees></Position><AltitudeMeters>79.927</AltitudeMeters><DistanceMeters>14238.382</DistanceMeters><Cadence>76</Cadence><Extensions><TPX xmlns=\"http://www.garmin.com/xmlschemas/ActivityExtension/v2\"><Watts>66</Watts></TPX></Extensions></Trackpoint><Trackpoint><Time>2008-03-03T23:11:22Z</Time><Position><LatitudeDegrees>35.863475</LatitudeDegrees><LongitudeDegrees>-78.899146</LongitudeDegrees></Position><AltitudeMeters>79.446</AltitudeMeters><DistanceMeters>14248.812</DistanceMeters><Cadence>79</Cadence><Extensions><TPX xmlns=\"http://www.garmin.com/xmlschemas/ActivityExtension/v2\"><Watts>60</Watts></TPX></Extensions></Trackpoint><Trackpoint><Time>2008-03-03T23:11:23Z</Time><Position><LatitudeDegrees>35.863457</LatitudeDegrees><LongitudeDegrees>-78.899261</LongitudeDegrees></Position><AltitudeMeters>79.446</AltitudeMeters><DistanceMeters>14259.354</DistanceMeters><Cadence>80</Cadence><Extensions><TPX xmlns=\"http://www.garmin.com/xmlschemas/ActivityExtension/v2\"><Watts>60</Watts></TPX></Extensions></Trackpoint><Trackpoint><Time>2008-03-03T23:11:24Z</Time><Position><LatitudeDegrees>35.863439</LatitudeDegrees><LongitudeDegrees>-78.899379</LongitudeDegrees></Position><AltitudeMeters>78.485</AltitudeMeters><DistanceMeters>14270.209</DistanceMeters><Cadence>81</Cadence><Extensions><TPX xmlns=\"http://www.garmin.com/xmlschemas/ActivityExtension/v2\"><Watts>60</Watts></TPX></Extensions></Trackpoint><Trackpoint><Time>2008-03-03T23:11:25Z</Time><Position><LatitudeDegrees>35.863421</LatitudeDegrees><LongitudeDegrees>-78.899500</LongitudeDegrees></Position><AltitudeMeters>78.485</AltitudeMeters><DistanceMeters>14281.277</DistanceMeters><Cadence>84</Cadence><Extensions><TPX xmlns=\"http://www.garmin.com/xmlschemas/ActivityExtension/v2\"><Watts>68</Watts></TPX></Extensions></Trackpoint><Trackpoint><Time>2008-03-03T23:11:26Z</Time><Position><LatitudeDegrees>35.863403</LatitudeDegrees><LongitudeDegrees>-78.899623</LongitudeDegrees></Position><AltitudeMeters>77.523</AltitudeMeters><DistanceMeters>14292.605</DistanceMeters><Cadence>85</Cadence><Extensions><TPX xmlns=\"http://www.garmin.com/xmlschemas/ActivityExtension/v2\"><Watts>69</Watts></TPX></Extensions></Trackpoint><Trackpoint><Time>2008-03-03T23:11:27Z</Time><Position><LatitudeDegrees>35.863383</LatitudeDegrees><LongitudeDegrees>-78.899748</LongitudeDegrees></Position><AltitudeMeters>77.523</AltitudeMeters><DistanceMeters>14304.128</DistanceMeters><Cadence>87</Cadence><Extensions><TPX 
